vi "Untitled 5 (SubVI).vi"(10 "Numeric in":i32, 11 "dt (ms)":u32) -> (3 "Numeric out":dbl)   [LabVIEW 2016]
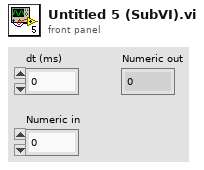
[diagram p1: front panel]
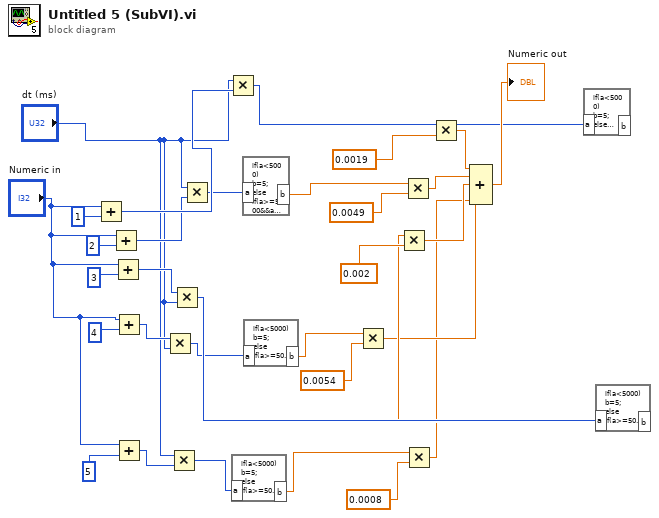
[diagram p0: block diagram]
diagram:
  n1 = Add(x="Numeric in", y=1) -> (x+y=w22:i32)
  n2 = Add(x="Numeric in", y=2) -> (x+y=w19:i32)
  n3 = Add(x="Numeric in", y=3 ("x")) -> (x+y=w16:i32)
  n4 = Add(x="Numeric in", y=4 ("x")) -> (x+y=w13:i32)
  n5 = Add(x="Numeric in", y=5 ("x")) -> (x+y=w6:i32)
  n6 = Multiply(x=w13, y="dt (ms)") -> (x*y=w12:u32)
  n7 = Multiply(x="dt (ms)", y=w6) -> (x*y=w4:u32)
  n8 = Multiply(x=w16, y="dt (ms)") -> (x*y=w17:u32)
  n9 = Multiply(x="dt (ms)", y=w19) -> (x*y=w20:u32)
  n10 = Multiply(x="dt (ms)", y=w22) -> (x*y=w23:u32)
  n11 = formula code="if(a<5000)\nb=5;\nelse \nif(a>=5000&&a<13000)\nb=9;\nelse\nif(a>=13000&&a<18000)\nb=13;\nelse\nif(a>=18000&&a<23000)\nb=7;\nelse\nif(a>=23000&&a<33000)\nb=-8;\nelse\nif(a>=33000)\nb=0;"("a"=w4) -> ("b"=w2:dbl)
  n12 = formula code="if(a<5000)\nb=5;\nelse \nif(a>=5000&&a<13000)\nb=9;\nelse\nif(a>=13000&&a<18000)\nb=13;\nelse\nif(a>=18000&&a<23000)\nb=7;\nelse\nif(a>=23000&&a<33000)\nb=-8;\nelse\nif(a>=33000)\nb=0;"("a"=w20) -> ("b"=w18:dbl)
  n13 = formula code="if(a<5000)\nb=5;\nelse \nif(a>=5000&&a<13000)\nb=9;\nelse\nif(a>=13000&&a<18000)\nb=13;\nelse\nif(a>=18000&&a<23000)\nb=7;\nelse\nif(a>=23000&&a<33000)\nb=-8;\nelse\nif(a>=33000)\nb=0;"("a"=w12) -> ("b"=w11:dbl)
  n14 = Multiply(x=w11, y=0.0054) -> (x*y=w9:dbl)
  n15 = Multiply(x=w18, y=0.0049) -> (x*y=w31:dbl)
  n16 = Multiply(x=w2, y=0.0008) -> (x*y=w1:dbl)
  n17 = formula code="if(a<5000)\nb=5;\nelse \nif(a>=5000&&a<13000)\nb=9;\nelse\nif(a>=13000&&a<18000)\nb=13;\nelse\nif(a>=18000&&a<23000)\nb=7;\nelse\nif(a>=23000&&a<33000)\nb=-8;\nelse\nif(a>=33000)\nb=0;"("a"=w23) -> ("b"=w21:dbl)
  n18 = Multiply(x=w21, y=0.0019) -> (x*y=w30:dbl)
  n19 = formula code="if(a<5000)\nb=5;\nelse \nif(a>=5000&&a<13000)\nb=9;\nelse\nif(a>=13000&&a<18000)\nb=13;\nelse\nif(a>=18000&&a<23000)\nb=7;\nelse\nif(a>=23000&&a<33000)\nb=-8;\nelse\nif(a>=33000)\nb=0;"("a"=w17) -> ("b"=w15:dbl)
  n20 = Multiply(x=w15, y=0.002) -> (x*y=w32:dbl)
  n21 = Compound Arithmetic op=ADD(w30, w31, w32, w9, w1) -> (→"Numeric out":dbl)
